vi "Diode-Time-Zero.vi"(8 "error in (no error)":errorcluster, 11 "connection ID":refnum<k5>) -> (0 "error out":errorcluster, 3 "connection ID out":refnum<k5>)   [LabVIEW 2020]
panel:
  # "Diode to Time Zero"
  # "Resets trigger count and updates real-time clock on the STM32 diode."
  # "Input an already-opened TCP connection."
  # "Concrete actions:\n1. Set trigger count to zero.\n2. Set current time on diode according to this system's clock."
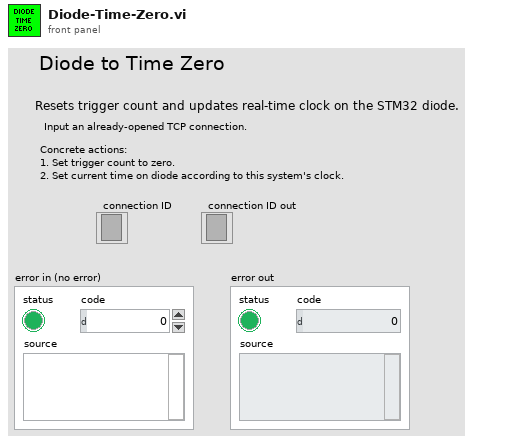
[diagram p1: front panel]
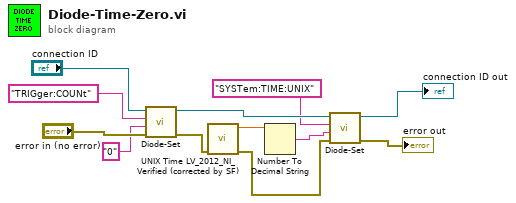
[diagram p0: block diagram]
diagram:
  n1 = call "Diode-Set.vi"("error in (no error)"="error in (no error)", "Set Value"="0", "Diode Keyword (leave off space, value)"="TRIGger:COUNt", "connection ID"="connection ID") -> ("error out"=w5:errorcluster, "connection ID out"=w11:refnum<k5>)  [unwired: 6 in]
  n2 = call "UNIX Time LV_2012_NI_Verified (corrected by SF).vi"("error in (no error)"=w5) -> ("error out"=w6:errorcluster, "Unix time"=w7:dbl)  [unwired: 9 in]
  n3 = Number To Decimal String(number=w7) -> (decimal integer string=w8:string)  [unwired: 1 in]
  n4 = call "Diode-Set.vi"("error in (no error)"=w6, "Set Value"=w8, "Diode Keyword (leave off space, value)"="SYSTem:TIME:UNIX", "connection ID"=w11) -> ("error out"=→"error out":errorcluster, "connection ID out"=→"connection ID out":refnum<k5>)  [unwired: 6 in]
